vi "HEWH RLT Read Single Channel.vi"(8 "Error In":errorcluster, 10 "all rows":string[](array[string]), 11 "Panel In":T1[](array[typedef])) -> (0 "Error Out":errorcluster, 3 "Panel Out":T1[](array[typedef]))   [LabVIEW 2016]
uses:
  Type Definitions/HEWH Channel Label RLT.ctl
  Custom Instrument Control/MW100/Type Definitions/Station ID Selector.ctl
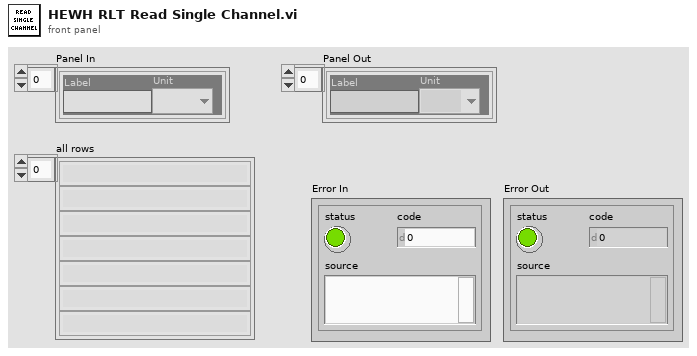
[diagram p1: front panel]
types:
  T1 = typedef "HEWH Channel Label RLT.ctl" = cluster{"Label":string, "Unit":T2}
  T2 = typedef "Station ID Selector.ctl" = enum16{"", "A", "B", "C", "D", "Global"}
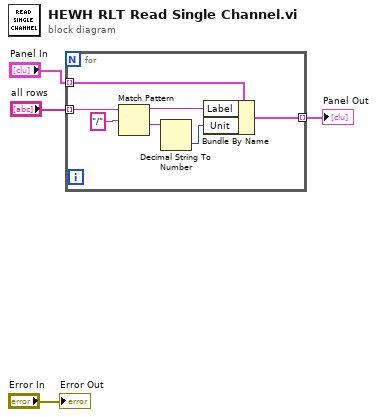
[diagram p0: block diagram]
diagram:
  n1 = for {
    tunnel: "Panel In" -> [w9] mode=indexing
    tunnel: "all rows" -> [w11] mode=indexing
    tunnel: [w6] -> w4 mode=indexing
    n2 = Match Pattern(string=w11, regular expression="/") -> (before substring=w8:string, after substring=w7:string)  [unwired: 1 in, 2 out]
    n3 = Decimal String To Number(string=w7) -> (number=w5:i32)  [unwired: 2 in, 1 out]
    n4 = Bundle By Name(cluster=w9, "Label"=w8, "Unit"=w5) -> (w6:T1)
  }
  "Panel Out" <- w4
  "Error Out" <- "Error In"
